vi "RichToFlatgoogle_protobuf_Type.vi"(5 "OutputClusterType":T1, 11 "InputCluster":T9) -> (3 "OutputCluster":T1)   [LabVIEW 2021, in "ni.measurementlink.measurement.v2.api.lvlib"]
uses:
  ni.measurementlink.measurement.v2.api.lvlib
  google_protobuf_Type.ctl
  google_protobuf_Field.ctl
  google_protobuf_Field_Kind.ctl
  google_protobuf_Field_Cardinality.ctl
  google_protobuf_Option.ctl
  google_protobuf_Any.ctl
  google_protobuf_SourceContext.ctl
  google_protobuf_Syntax.ctl
  google_protobuf_Type_Flat.ctl
  google_protobuf_Field_Flat.ctl
  google_protobuf_Option_Flat.ctl
  google_protobuf_Any_Flat.ctl
  google_protobuf_SourceContext_Flat.ctl
  RichToFlatgoogle_protobuf_Any.vi
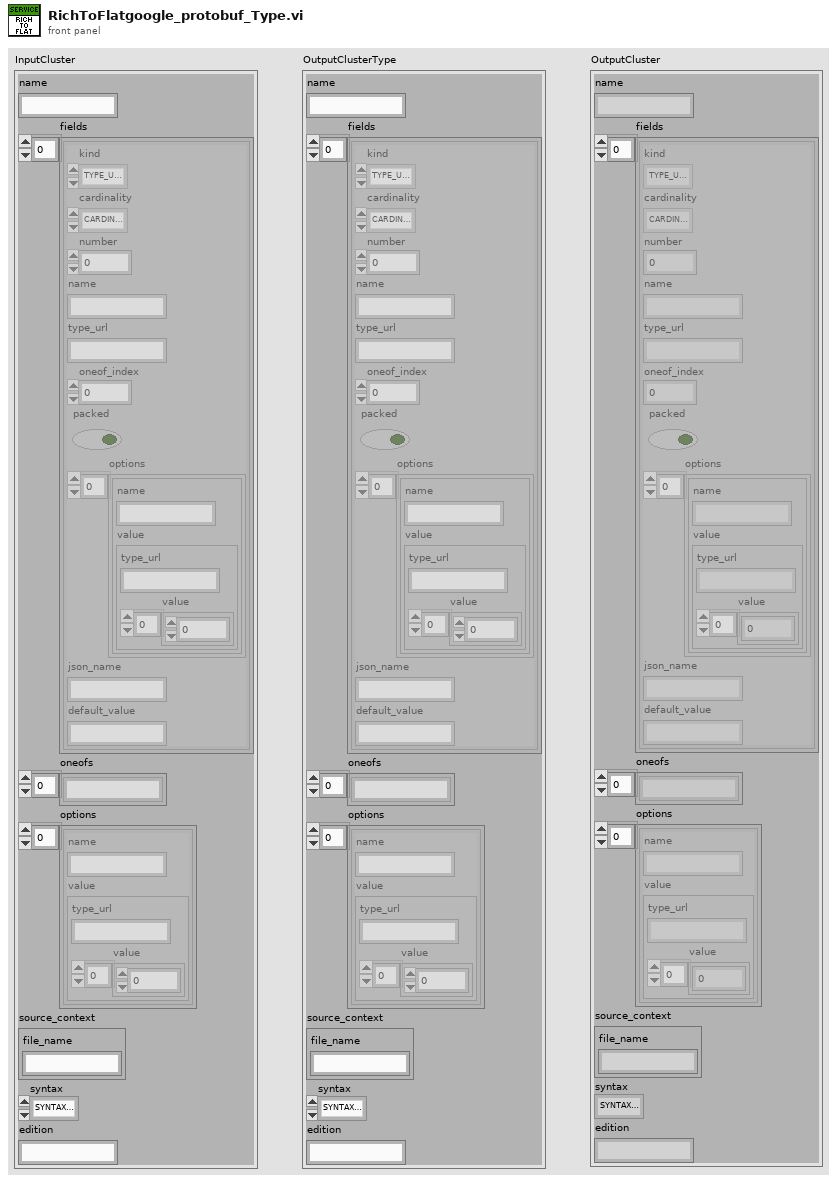
[diagram p1: front panel]
types:
  T1 = typedef "ni.measurementlink.measurement.v2.api.lvlib/google_protobuf_Type_Flat.ctl" = cluster{"name":string, "fields":T2[], "oneofs":string[], "options":T5[], "source_context":T7, "syntax":T8, "edition":string}
  T2 = typedef "ni.measurementlink.measurement.v2.api.lvlib/google_protobuf_Field_Flat.ctl" = cluster{"kind":T3, "cardinality":T4, "number":i32, "name":string, "type_url":string, "oneof_index":i32, "packed":bool, "options":T5[], "json_name":string, "default_value":string}
  T3 = typedef "ni.measurementlink.measurement.v2.api.lvlib/google_protobuf_Field_Kind.ctl" = enum32{"TYPE_UNKNOWN", "TYPE_DOUBLE", "TYPE_FLOAT", "TYPE_INT64", "TYPE_UINT64", "TYPE_INT32", "TYPE_FIXED64", "TYPE_FIXED32", "TYPE_BOOL", "TYPE_STRING", "TYPE_GROUP", "TYPE_MESSAGE", "TYPE_BYTES", "TYPE_UINT32", "TYPE_ENUM", "TYPE_SFIXED32", "TYPE_SFIXED64", "TYPE_SINT32", "TYPE_SINT64"}
  T4 = typedef "ni.measurementlink.measurement.v2.api.lvlib/google_protobuf_Field_Cardinality.ctl" = enum32{"CARDINALITY_UNKNOWN", "CARDINALITY_OPTIONAL", "CARDINALITY_REQUIRED", "CARDINALITY_REPEATED"}
  T5 = typedef "ni.measurementlink.measurement.v2.api.lvlib/google_protobuf_Option_Flat.ctl" = cluster{"name":string, "value":T6}
  T6 = typedef "ni.measurementlink.measurement.v2.api.lvlib/google_protobuf_Any_Flat.ctl" = cluster{"type_url":string, "value":u8[]}
  T7 = typedef "ni.measurementlink.measurement.v2.api.lvlib/google_protobuf_SourceContext_Flat.ctl" = cluster{"file_name":string}
  T8 = typedef "ni.measurementlink.measurement.v2.api.lvlib/google_protobuf_Syntax.ctl" = enum32{"SYNTAX_PROTO2", "SYNTAX_PROTO3", "SYNTAX_EDITIONS"}
  T9 = typedef "ni.measurementlink.measurement.v2.api.lvlib/google_protobuf_Type.ctl" = cluster{"name":string, "fields":T10[], "oneofs":string[], "options":T11[], "source_context":T13, "syntax":T8, "edition":string}
  T10 = typedef "ni.measurementlink.measurement.v2.api.lvlib/google_protobuf_Field.ctl" = cluster{"kind":T3, "cardinality":T4, "number":i32, "name":string, "type_url":string, "oneof_index":i32, "packed":bool, "options":T11[], "json_name":string, "default_value":string}
  T11 = typedef "ni.measurementlink.measurement.v2.api.lvlib/google_protobuf_Option.ctl" = cluster{"name":string, "value":T12}
  T12 = typedef "ni.measurementlink.measurement.v2.api.lvlib/google_protobuf_Any.ctl" = cluster{"type_url":string, "value":u8[]}
  T13 = typedef "ni.measurementlink.measurement.v2.api.lvlib/google_protobuf_SourceContext.ctl" = cluster{"file_name":string}
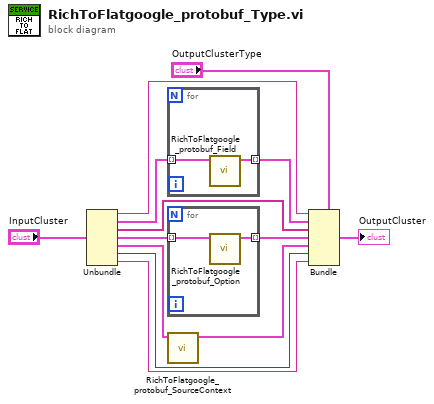
[diagram p0: block diagram]
diagram:
  n1 = Unbundle "Unbundle"("InputCluster") -> ("name"=w10:string, "fields"=w9:T10[], "oneofs"=w7:string[], "options"=w6:T11[], "source_context"=w4:T13, "syntax"=w2:T8, "edition"=w1:string)
  n2 = for {
    tunnel: w9 -> [w15] mode=indexing
    tunnel: [w14] -> w8 mode=indexing
    n3 = call "RichToFlatgoogle_protobuf_Field.vi"("InputCluster"=w15) -> ("OutputCluster"=w14:T2)  [unwired: 10 in]
  }
  n4 = for {
    tunnel: w6 -> [w17] mode=indexing
    tunnel: [w16] -> w5 mode=indexing
    n5 = call "RichToFlatgoogle_protobuf_Option.vi"("InputCluster"=w17) -> ("OutputCluster"=w16:T5)  [unwired: 10 in]
  }
  n6 = call "RichToFlatgoogle_protobuf_SourceContext.vi"("InputCluster"=w4) -> ("OutputCluster"=w3:T7)  [unwired: 10 in]
  n7 = Bundle "Bundle"(cluster="OutputClusterType", "name"=w10, "fields"=w8, "oneofs"=w7, "options"=w5, "source_context"=w3, "syntax"=w2, "edition"=w1) -> (→"OutputCluster":T1)
